vi "DecimalToRGB.vi"(0 "DecRGB":u32) -> (2 "Red":u8, 3 "Green":u8, 4 "Blue":u8)   [LabVIEW 2021]
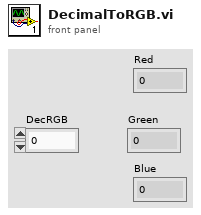
[diagram p1: front panel]
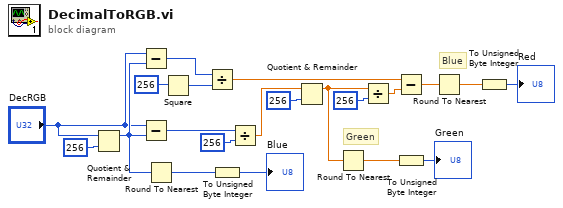
[diagram p0: block diagram]
diagram:
  # "Blue"
  # "Green"
  n1 = Quotient & Remainder(x="DecRGB", y=u32 256 ("x")) -> (x-y*floor(x/y)=w10:u32)  [unwired: 1 out]
  n2 = Subtract(x="DecRGB", y=w10) -> (x-y=w14:u32)
  n3 = Subtract(x="DecRGB", y=w10) -> (x-y=w19:u32)
  n4 = Round To Nearest(number=w10) -> (nearest integer value=w6:u32)
  n5 = Square(x=u32 256 ("y")) -> (x^2=w15:u32)
  n6 = Divide(x=w14, y=w15) -> (x/y=w12:dbl)
  n7 = To Unsigned Byte Integer(number=w6) -> (unsigned 8bit integer=→"Blue":u8)
  n8 = Divide(x=w19, y=u32 256) -> (x/y=w17:dbl)
  n9 = Quotient & Remainder(x=w17, y=u32 256 ("x")) -> (x-y*floor(x/y)=w9:dbl)  [unwired: 1 out]
  n10 = Round To Nearest(number=w9) -> (nearest integer value=w2:dbl)
  n11 = Divide(x=w9, y=u32 256 ("x")) -> (x/y=w11:dbl)
  n12 = Subtract(x=w12, y=w11) -> (x-y=w8:dbl)
  n13 = To Unsigned Byte Integer(number=w2) -> (unsigned 8bit integer=→"Green":u8)
  n14 = Round To Nearest(number=w8) -> (nearest integer value=w1:dbl)
  n15 = To Unsigned Byte Integer(number=w1) -> (unsigned 8bit integer=→"Red":u8)
